vi "CALC_EQU_STAT.vi"(0 "VISA IN":refnum<visa-resource-name>, 1 "Equation ON/OFF":bool, 5 "error in":errorcluster, 7 "Channel":i32) -> (14 "VISA Out":refnum<visa-resource-name>, 19 "error out":errorcluster)   [LabVIEW 2018, in "PNA-X.lvlib"]
doc: "CALCulate<cnum>:EQUation:STATe <bool> \n(Read-Write) Turns ON and OFF the equation on selected measurement for the specified channel. If \nthe equation is not valid, then processing is not performed. Use CALC:EQUation:VALid? to ensure \nthat the equation is valid. \nSee Critical Note \nParameters \n<cnum> Channel number of the measurement. There must be a selected measurement \non that channel. If unspecified, <cnum> is set to 1. \n<bool> ON (or 1) - turns equation ON. \nOFF (or 0) - turns equation OFF. \nExamples CALC:EQU:STAT 1 \ncalculate2:equation:state 0 \nQuery Syntax CALCulate<cnum>:EQUation:STATe? \n1503\n\nReturn Type Boolean \nDefault OFF (0)"
uses:
  PNA-X.lvlib
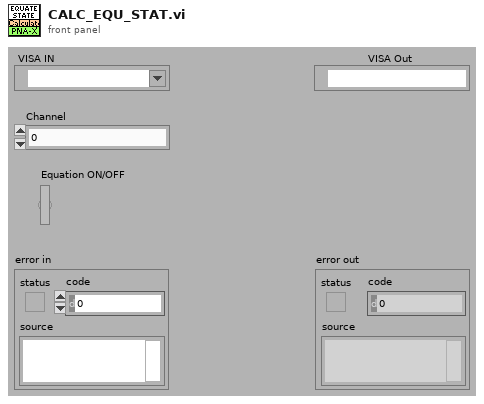
[diagram p1: front panel]
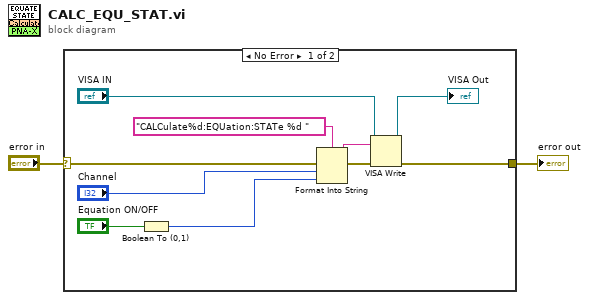
[diagram p0: block diagram]
diagram:
  n1 = case shown="No Error" "error in" {
    selector: "error in" -> [w12 w13]
    tunnel: [w7 w13] -> w1
    frame No Error {
      n2 = Boolean To (0,1)(Boolean="Equation ON/OFF") -> (0, 1=w3:i16)
      n3 = Format Into String(format string="CALCulate%d:EQUation:STATe %d " ("Cmdline"), error in=w12, "Channel", w3) -> (resulting string=w10:string, error out=w11:errorcluster)  [unwired: 1 in]
      n4 = VISA Write(VISA resource name="VISA IN", write buffer=w10, error in (no error)=w11) -> (VISA resource name out=→"VISA Out":refnum<visa-resource-name>, error out=w7:errorcluster)  [unwired: 1 out]
    }
    frame Error {
    }
  }
  "error out" <- w1
